vi "STM Get Connection Reference.vi"   [LabVIEW 2015, in "J1939 Addon Shared.lvlib"]
doc: "Returns the connection reference of the STM session."
uses:
  J1939 Addon Shared.lvlib
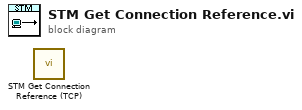
[diagram p0: block diagram]
diagram:
  n1 = call "STM Get Connection Reference (TCP).vi"() -> ()  [unwired: 9 in, 3 out]
